vi "File Viewer v4.vi"() -> ()   [LabVIEW 2019]
uses:
  <vilib>/Utility/file.llb/Read Delimited Spreadsheet (I64).vi
  <vilib>/Utility/file.llb/Write Delimited Spreadsheet (DBL).vi
panel:
  in  "Stop":bool
  in  "Tab Control":T1(tab)
  in  "update":bool
  out "Raw Image From Camera":i32[][](graph)
  in  "File Path for Image:":path
  out "Expected position on spectrometer (pixels):":dbl
  in  "Grating:":u16(ring) items=["Shimadzu 30-006  "]
  in  "Laser:":u16(ring) items=["800nm  "]
  in  "Harmonic":dbl min=10.0 max=40.0
  out "l (nm)":dbl
  out "E (J)":dbl
  out "E (eV)":dbl
  out "Nearest Harmonic of 800nm":dbl
  out "Vertical Binned Waveform Graph":i64[](graph)
  out "Cursor Position (pixels)":dbl
  out "Distance to nearest harmonic of 800nm (pixels)":dbl
  in  "Caibration Date":u16(ring) items=["first calibration - 7/31", "7/31-current"]
  in  "Correct for QE?":bool
  in  "Save text file":bool
  in  "Graph to export:":u16(ring) items=["Wavelength Graph", "Energy Graph", "Harmonics Graph"]
  out "Wavelength Graph":T2(graph)
  out "Energy Graph (eV)":cluster{"eV":dbl, "QE scaled count":dbl}[](graph)
  out "Harmonics Graph":cluster{dbl, "QE scaled count":dbl}[](graph)
  in  "Pump/Probe Run Folder:":path
  out "Distance to nearest harmonic of 800nm (pixels)":dbl
  out "Cursor Position on CCD  (pixels)":dbl
  out "Nearest Harmonic of 800nm":dbl
  out "E (eV) 2":dbl
  out "E (J)":dbl
  out "l (nm)":dbl
  in  "Pump/Probe Harmonic:":dbl min=10.0 max=40.0
  out "Expected position on spectrometer (pixels):":dbl
  out "Time delay":dbl
  out "XUV":dbl[][](graph)
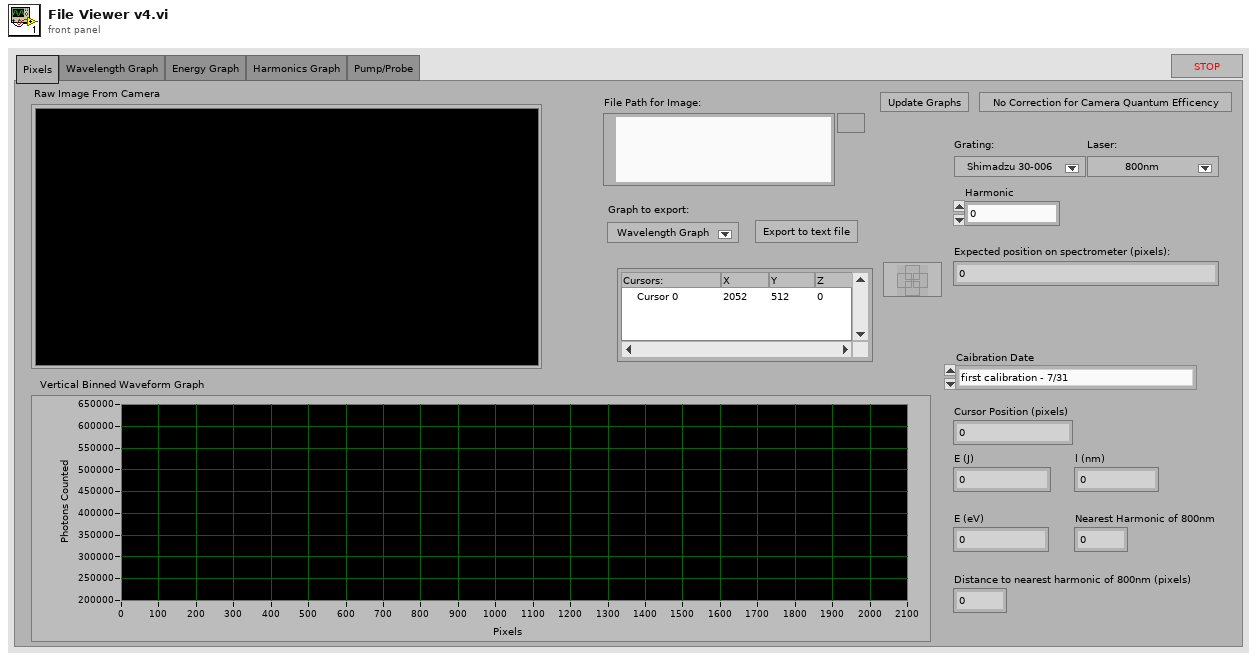
[diagram p1: front panel]
types:
  T1 = enum32{"Pixels", "Wavelength Graph", "Energy Graph", "Harmonics Graph", "Pump/Probe"}
  T2 = cluster{"No prefix":dbl, "QE scaled count":dbl}[]
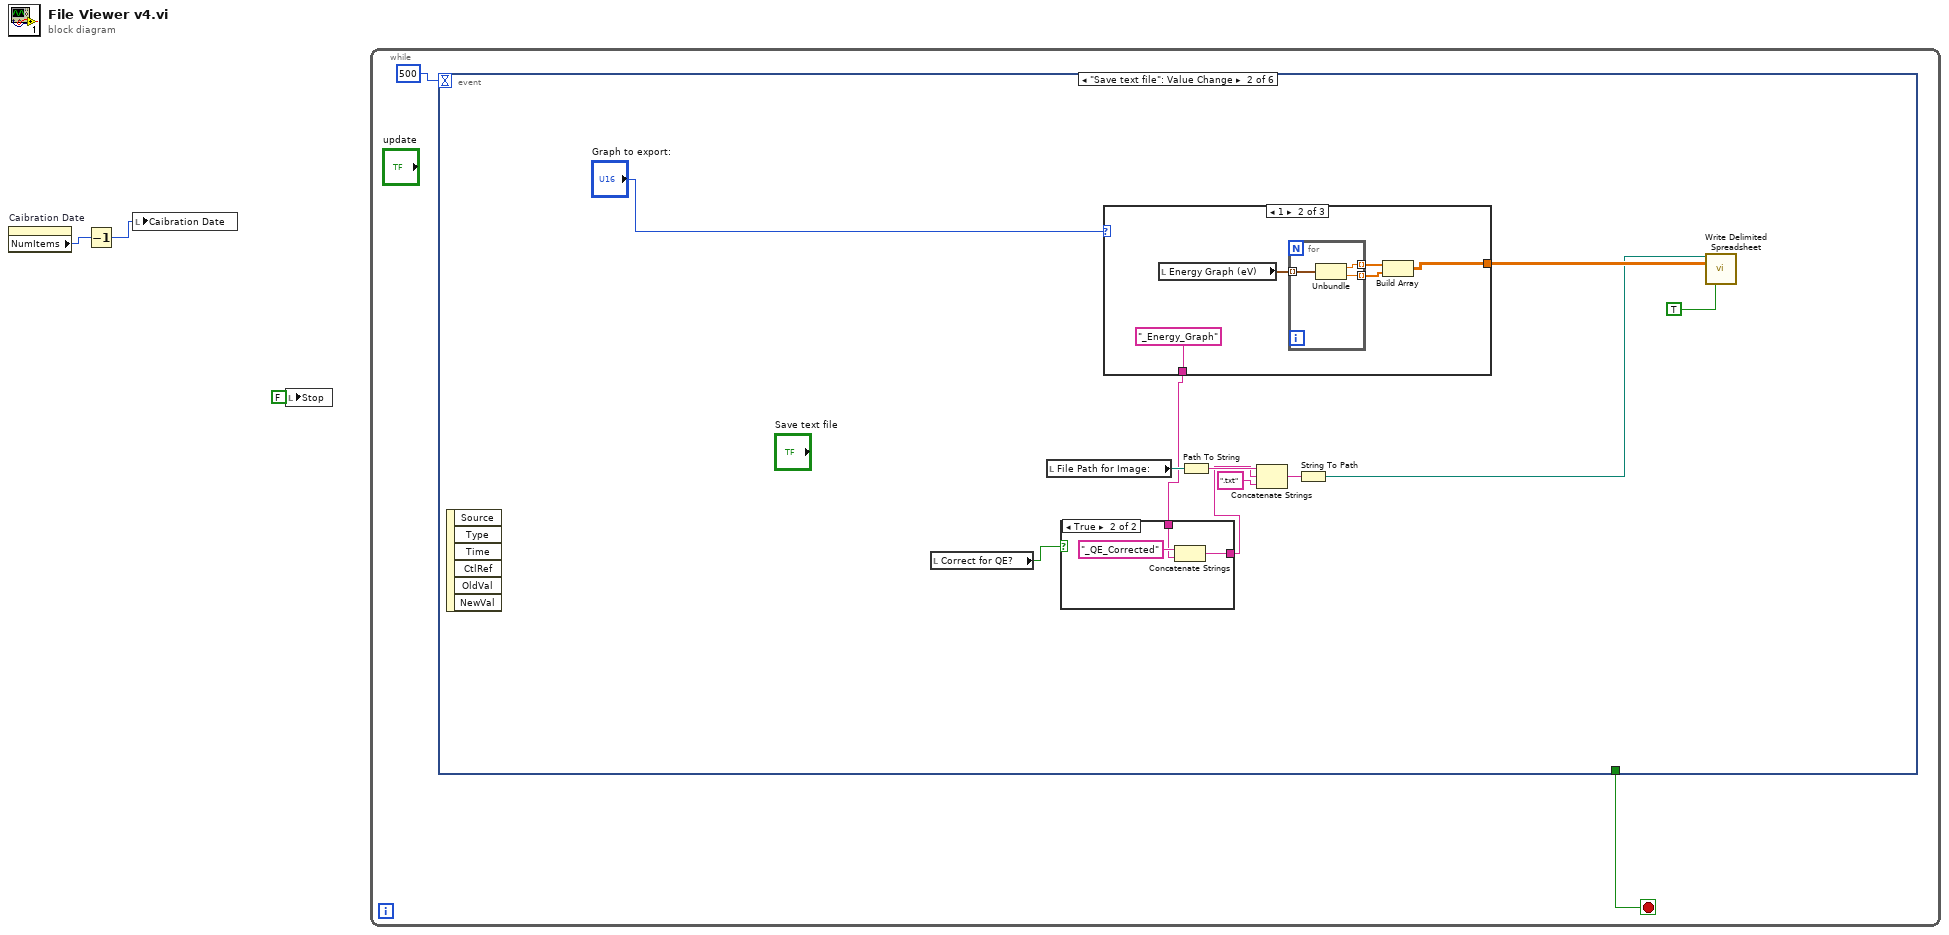
[diagram p0: block diagram]
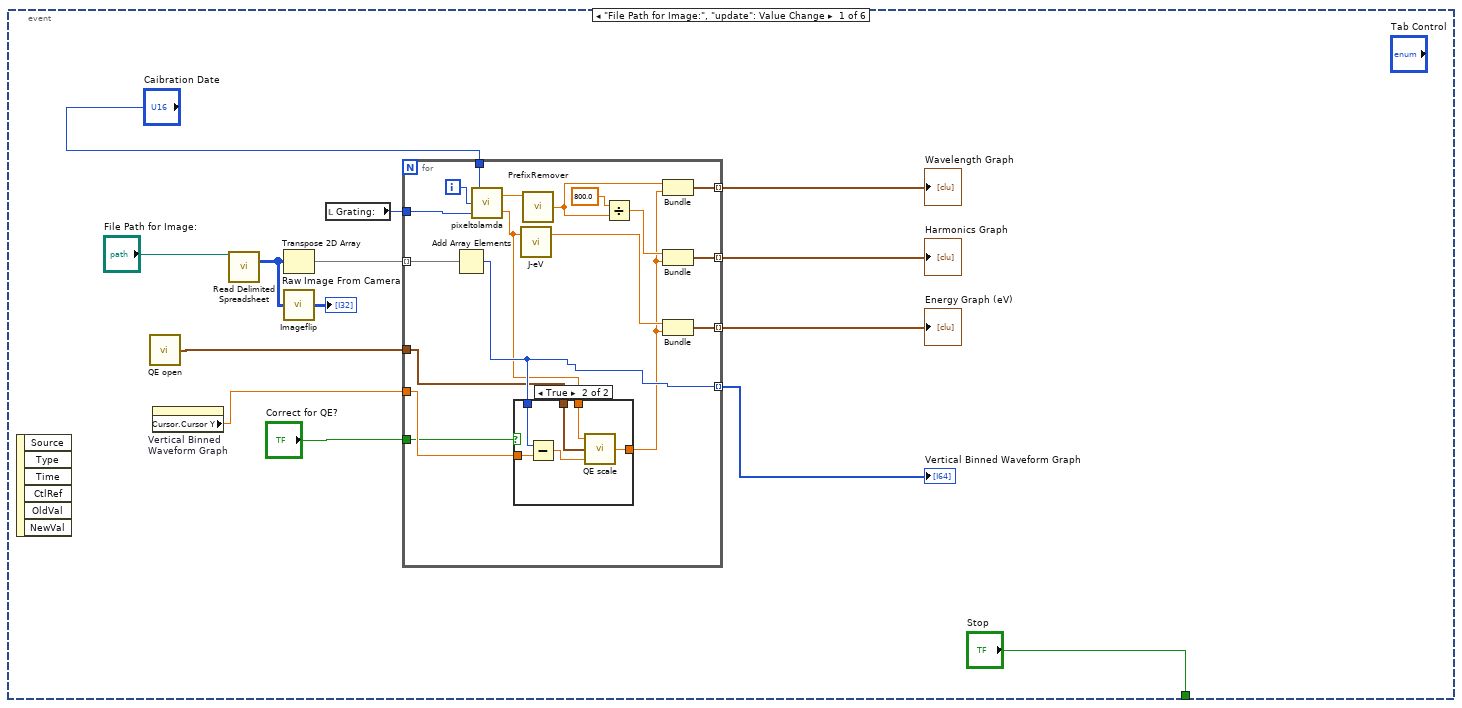
[diagram p2: hidden frame]
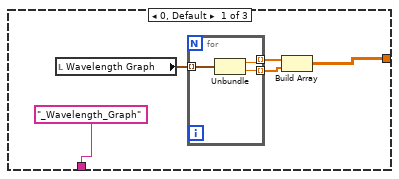
[diagram p5: hidden frame]
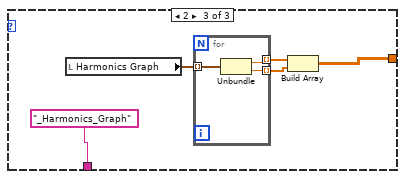
[diagram p6: hidden frame]
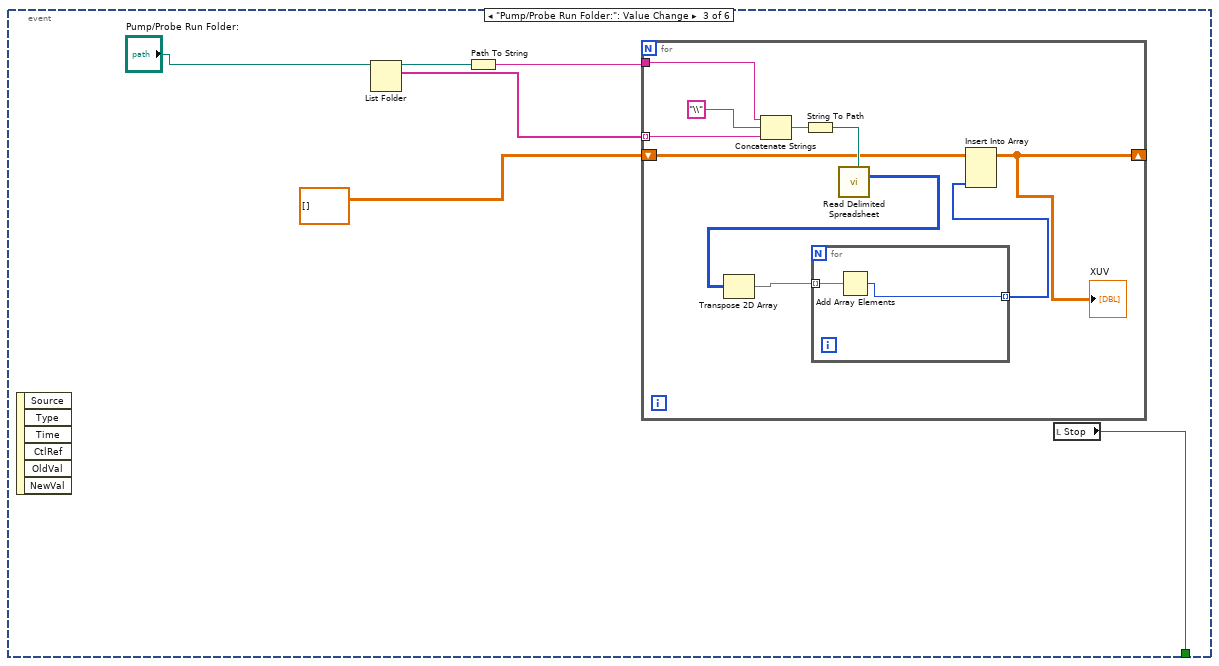
[diagram p7: hidden frame]
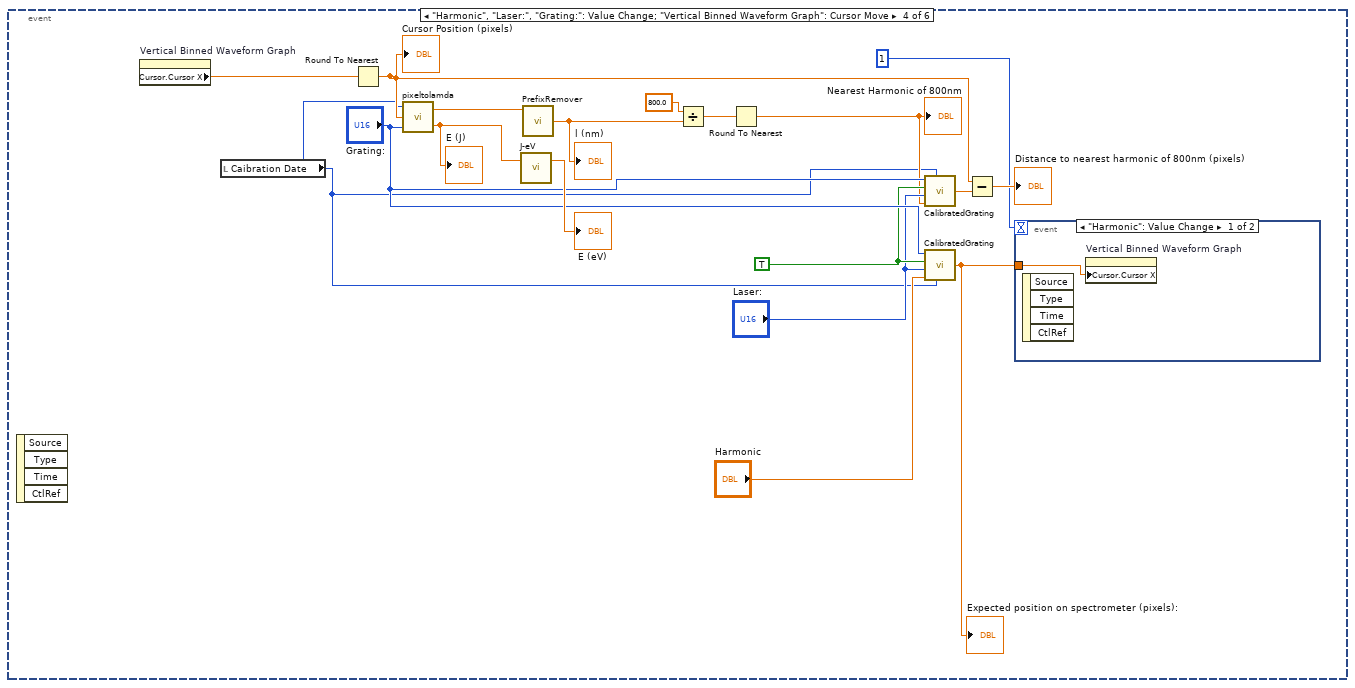
[diagram p8: hidden frame]
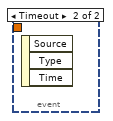
[diagram p9: hidden frame]
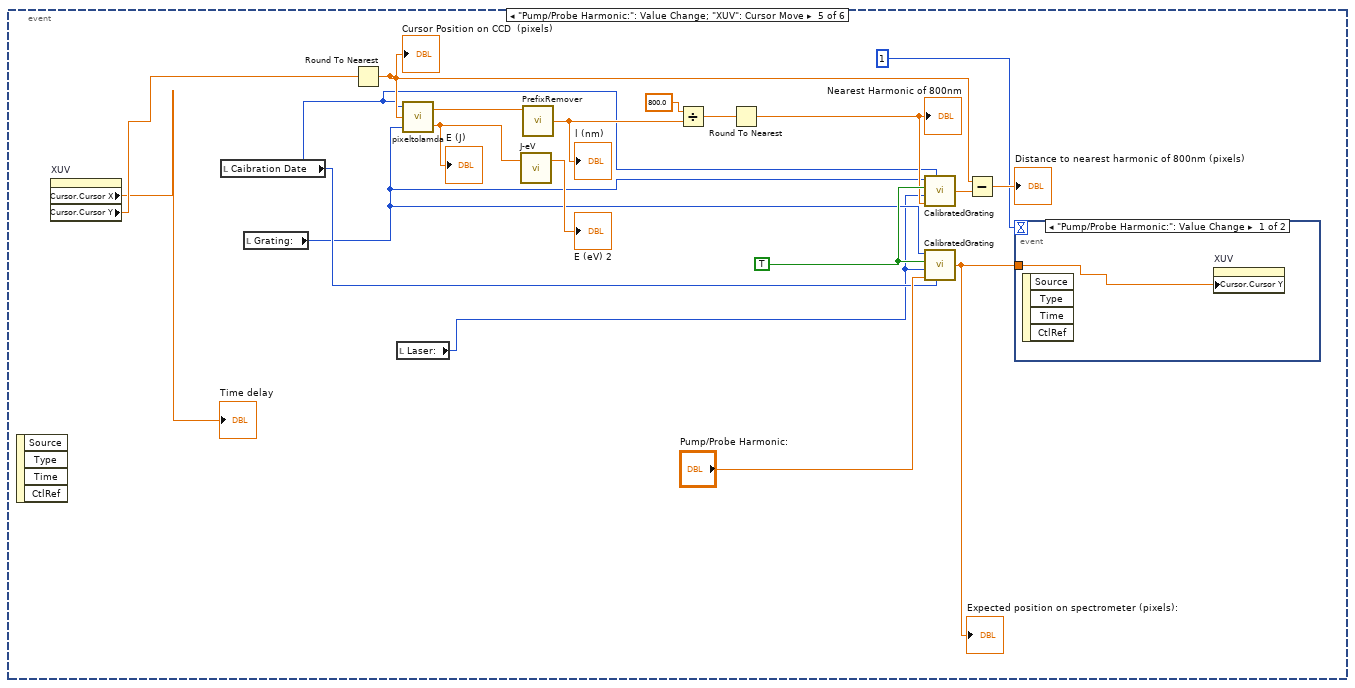
[diagram p10: hidden frame]
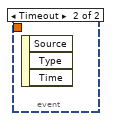
[diagram p11: hidden frame]
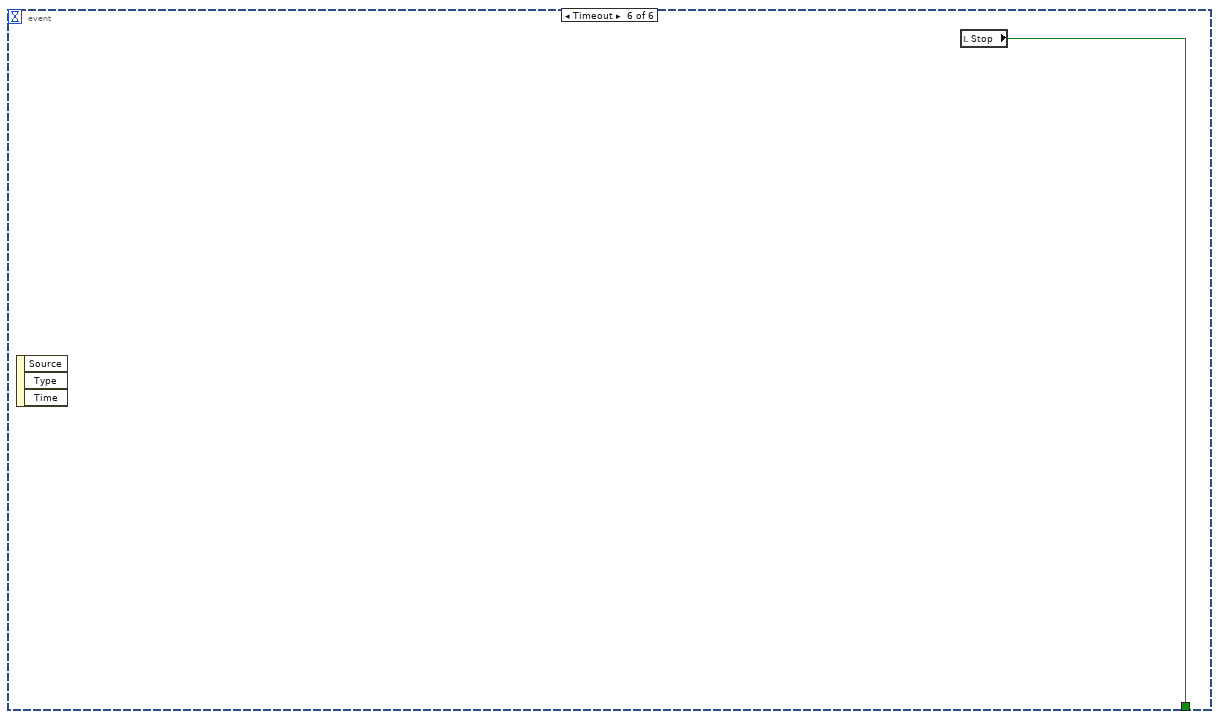
[diagram p12: hidden frame]
diagram:
  n1 = property on="Caibration Date" class="Ring (strict)"() -> ("NumItems"=w1:u32)  [unwired: 2 in, 2 out]
  n2 = Decrement(x=w1) -> (x-1=w2:u32)
  n3 = local write "Caibration Date"(w2) -> ()
  n4 = local write "Stop"(FALSE) -> ()
  n5 = while {
    stop <- w5 stop-if-true
    n6 = event shown="[1] \"Save text file\": Value Change" {
      selector: _ -> [_ _ _ _ _ _]
      dyn-events: _ -> [_ _ _ _ _ _]
      timeout: 500 -> [_ _ _ _ _ _]
      tunnel: ["Stop" _ w85 _ _ w141] -> w5
      event "File Path for Image:", "update": Value Change {
        n7 = event-data() -> ()  [unwired: 1 in, 6 out]
        n8 = call "QE open.vi"() -> ("QE data"=w8:cluster{"Numeric":dbl, dbl}[])
        n9 = property on="Vertical Binned Waveform Graph" class="WFGraph (strict)"() -> ("Cursor.Cursor Y"=w7:dbl)  [unwired: 2 in, 2 out]
        n10 = call-poly <vilib>:"Read Delimited Spreadsheet.vi"("file path (dialog if empty)"="File Path for Image:") -> ("all rows"=w16:i64[][])  [unwired: 9 in, 5 out]
        n11 = Transpose 2D Array(2D array=w16) -> (transposed array=w15:i64[][])
        n12 = call "Imageflip.vi"("2D array"=w16) -> ("transposed array"=→"Raw Image From Camera":i32[][])
        n13 = local read "Grating:"() -> (w13:u16)
        n14 = for {
          tunnel: w15 -> [w37] mode=indexing
          tunnel: [w25] -> w14 mode=indexing
          tunnel: w13 -> [w35]
          tunnel: [w34] -> w12 mode=indexing
          tunnel: [w33] -> w11 mode=indexing
          tunnel: [w28] -> w10 mode=indexing
          tunnel: "Caibration Date" -> [w27]
          tunnel: w8 -> [w24]
          tunnel: w7 -> [w26]
          tunnel: "Correct for QE?" -> [w21]
          i -> [w36]
          n15 = Add Array Elements(numeric array=w37) -> (sum=w25:i64)
          n16 = call "pixeltolamda.vi"("Grating:"=w35, "Pixel Postion"=w36, "Caibration Date"=w27) -> ("E (J)"=w20:dbl, "lamda (m)"=w31:dbl)
          n17 = case shown="True" w21 {
            tunnel: w26 -> [_ w44]
            tunnel: w25 -> [w38 w43]
            tunnel: w24 -> [_ w41]
            tunnel: w20 -> [_ w40]
            tunnel: [w38 w39] -> w22
            frame False {
            }
            frame True {
              n18 = Subtract(x=w43, y=w44) -> (x-y=w42:dbl)
              n19 = call "QE scale.vi"("Raw Photon Count"=w42, "QE data"=w41, "Energy (J)"=w40) -> ("QE scaled count"=w39:dbl)
            }
          }
          n20 = call "J-eV.vi"("J"=w20) -> ("eV"=w23:dbl)  [unwired: 1 in, 1 out]
          n21 = call "PrefixRemover.vi"("Nano"=w31) -> ("No prefix"=w30:dbl)  [unwired: 3 in]
          n22 = Divide(x=800.0, y=w30) -> (x/y=w29:dbl)
          n23 = Bundle("No prefix"=w30, "QE scaled count"=w22) -> (w34:cluster{"No prefix":dbl, "QE scaled count":dbl})  [unwired: 1 in]
          n24 = Bundle(w29, "QE scaled count"=w22) -> (w28:cluster{dbl, "QE scaled count":dbl})  [unwired: 1 in]
          n25 = Bundle("eV"=w23, "QE scaled count"=w22) -> (w33:cluster{"eV":dbl, "QE scaled count":dbl})  [unwired: 1 in]
        }
        "Vertical Binned Waveform Graph" <- w14
        "Wavelength Graph" <- w12
        "Energy Graph (eV)" <- w11
        "Harmonics Graph" <- w10
      }
      event "Save text file": Value Change {
        n26 = event-data() -> ()  [unwired: 1 in, 6 out]
        n27 = local read "Correct for QE?"() -> (w49:bool)
        n28 = local read "File Path for Image:"() -> (w52:path)
        n29 = case shown="1" "Graph to export:" {
          tunnel: [w61 w69 w77] -> w54
          tunnel: ["_Wavelength_Graph" ("pattern (all files)") "_Energy_Graph" ("pattern (all files)") "_Harmonics_Graph" ("pattern (all files)")] -> w47
          frame 0, Default {
            n30 = local read "Wavelength Graph"() -> (w64:T2)
            n31 = for {
              tunnel: w64 -> [w67] mode=indexing
              tunnel: [w66] -> w63 mode=indexing
              tunnel: [w65] -> w62 mode=indexing
              n32 = Unbundle(w67) -> ("No prefix"=w66:dbl, "QE scaled count"=w65:dbl)
            }
            n33 = Build Array(w63, w62) -> (w61:dbl[][])
          }
          frame 1 {
            n34 = local read "Energy Graph (eV)"() -> (w70:cluster{"eV":dbl, "QE scaled count":dbl}[])
            n35 = for {
              tunnel: w70 -> [w75] mode=indexing
              tunnel: [w74] -> w72 mode=indexing
              tunnel: [w73] -> w71 mode=indexing
              n36 = Unbundle(w75) -> ("eV"=w74:dbl, "QE scaled count"=w73:dbl)
            }
            n37 = Build Array(w72, w71) -> (w69:dbl[][])
          }
          frame 2 {
            n38 = local read "Harmonics Graph"() -> (w78:cluster{dbl, "QE scaled count":dbl}[])
            n39 = for {
              tunnel: w78 -> [w83] mode=indexing
              tunnel: [w82] -> w80 mode=indexing
              tunnel: [w81] -> w79 mode=indexing
              n40 = Unbundle(w83) -> (w82:dbl, "QE scaled count"=w81:dbl)
            }
            n41 = Build Array(w80, w79) -> (w77:dbl[][])
          }
        }
        n42 = case shown="True" w49 {
          tunnel: [w56 w58] -> w48
          tunnel: w47 -> [w56 w57]
          frame False {
          }
          frame True {
            n43 = Concatenate Strings("_QE_Corrected" ("pattern (all files)"), w57) -> (w58:string)
          }
        }
        n44 = Path To String(path=w52) -> (string=w51:string)
        n45 = Concatenate Strings(w51, w48, ".txt" ("pattern (all files)")) -> (w46:string)
        n46 = String To Path(string=w46) -> (path=w45:path)
        n47 = call-poly <vilib>:"Write Delimited Spreadsheet.vi"("file path (dialog if empty)"=w45, "2D data"=w54, "transpose? (no:F)"=TRUE) -> ()  [unwired: 11 in, 2 out]
      }
      event "Pump/Probe Run Folder:": Value Change {
        n48 = event-data() -> ()  [unwired: 1 in, 6 out]
        n49 = List Folder(path="Pump/Probe Run Folder:") -> (path out=w87:path, filenames=w88:string[])  [unwired: 3 in, 2 out]
        n50 = Path To String(path=w87) -> (string=w86:string)
        n51 = for {
          tunnel: w88 -> [w97] mode=indexing
          tunnel: w86 -> [w95]
          shift-right: [w90] -> _
          shift-left: dbl[][] [] -> [w94]
          n52 = Concatenate Strings(w95, "\\" ("string"), w97) -> (w99:string)
          n53 = String To Path(string=w99) -> (path=w98:path)
          n54 = call-poly <vilib>:"Read Delimited Spreadsheet.vi"("file path (dialog if empty)"=w98) -> ("all rows"=w92:i64[][])  [unwired: 9 in, 5 out]
          n55 = Transpose 2D Array(2D array=w92) -> (transposed array=w91:i64[][])
          n56 = for {
            tunnel: w91 -> [w101] mode=indexing
            tunnel: [w100] -> w93 mode=indexing
            n57 = Add Array Elements(numeric array=w101) -> (sum=w100:i64)
          }
          n58 = Insert Into Array(array=w94, new element=w93) -> (w90:dbl[][])  [unwired: 2 in]
          "XUV" <- w90
        }
        n59 = local read "Stop"() -> (w85:bool)
      }
      event "Harmonic", "Laser:", "Grating:": Value Change; "Vertical Binned Waveform Graph": Cursor Move {
        w111 = TRUE ("Subvi?")
        n60 = event-data() -> ()  [unwired: 1 in, 4 out]
        n61 = property on="Vertical Binned Waveform Graph" class="WFGraph (strict)"() -> ("Cursor.Cursor X"=w113:dbl)  [unwired: 2 in, 2 out]
        n62 = local read "Caibration Date"() -> (w102:u16)
        n63 = Round To Nearest(number=w113) -> (nearest integer value=w105:dbl)
        "Cursor Position (pixels)" <- w105
        n64 = call "pixeltolamda.vi"("Grating:"="Grating:", "Pixel Postion"=w105, "Caibration Date"=w102) -> ("E (J)"=w117:dbl, "lamda (m)"=w118:dbl)
        "E (J)" <- w117
        n65 = call "J-eV.vi"("J"=w117) -> ("eV"=→"E (eV)":dbl)  [unwired: 1 in, 1 out]
        n66 = call "PrefixRemover.vi"("Nano"=w118) -> ("No prefix"=w108:dbl)  [unwired: 3 in]
        "l (nm)" <- w108
        n67 = Divide(x=800.0, y=w108) -> (x/y=w115:dbl)
        n68 = Round To Nearest(number=w115) -> (nearest integer value=w109:dbl)
        "Nearest Harmonic of 800nm" <- w109
        n69 = call "CalibratedGrating.vi"("Grating:"="Grating:", "Subvi?"=w111, "Laser:"="Laser:", "Harmonic"=w109, "Caibration Date"=w102) -> ("Position on spectrometer (pixels):"=w107:dbl)
        n70 = call "CalibratedGrating.vi"("Grating:"="Grating:", "Subvi?"=w111, "Laser:"="Laser:", "Harmonic"="Harmonic", "Caibration Date"=w102) -> ("Position on spectrometer (pixels):"=w104:dbl)
        "Expected position on spectrometer (pixels):" <- w104
        n71 = Subtract(x=w105, y=w107) -> (x-y=→"Distance to nearest harmonic of 800nm (pixels)":dbl)
        n72 = event shown="[0] \"Harmonic\": Value Change" {
          selector: _ -> [_ _]
          dyn-events: _ -> [_ _]
          timeout: 1 -> [_ _]
          tunnel: w104 -> [w120 _]
          event "Harmonic": Value Change {
            n73 = event-data() -> ()  [unwired: 1 in, 4 out]
            n74 = property on="Vertical Binned Waveform Graph" class="WFGraph (strict)"("Cursor.Cursor X"=w120) -> ()  [unwired: 2 in, 2 out]
          }
          event Timeout {
            n75 = event-data() -> ()  [unwired: 1 in, 3 out]
          }
        }
      }
      event "Pump/Probe Harmonic:": Value Change; "XUV": Cursor Move {
        w133 = TRUE ("Subvi?")
        n76 = event-data() -> ()  [unwired: 1 in, 4 out]
        n77 = property on="XUV" class="IntGraph (strict)"() -> ("Cursor.Cursor X"=→"Time delay":dbl, "Cursor.Cursor Y"=w122:dbl)  [unwired: 2 in, 2 out]
        n78 = local read "Caibration Date"() -> (w125:u16)
        n79 = local read "Grating:"() -> (w124:u16)
        n80 = Round To Nearest(number=w122) -> (nearest integer value=w128:dbl)
        "Cursor Position on CCD  (pixels)" <- w128
        n81 = local read "Laser:"() -> (w123:u16)
        n82 = call "pixeltolamda.vi"("Grating:"=w124, "Pixel Postion"=w128, "Caibration Date"=w125) -> ("E (J)"=w137:dbl, "lamda (m)"=w138:dbl)
        "E (J)" <- w137
        n83 = call "J-eV.vi"("J"=w137) -> ("eV"=→"E (eV) 2":dbl)  [unwired: 1 in, 1 out]
        n84 = call "PrefixRemover.vi"("Nano"=w138) -> ("No prefix"=w131:dbl)  [unwired: 3 in]
        "l (nm)" <- w131
        n85 = Divide(x=800.0, y=w131) -> (x/y=w135:dbl)
        n86 = Round To Nearest(number=w135) -> (nearest integer value=w132:dbl)
        "Nearest Harmonic of 800nm" <- w132
        n87 = call "CalibratedGrating.vi"("Grating:"=w124, "Subvi?"=w133, "Laser:"=w123, "Harmonic"=w132, "Caibration Date"=w125) -> ("Position on spectrometer (pixels):"=w130:dbl)
        n88 = call "CalibratedGrating.vi"("Grating:"=w124, "Subvi?"=w133, "Laser:"=w123, "Harmonic"="Pump/Probe Harmonic:", "Caibration Date"=w125) -> ("Position on spectrometer (pixels):"=w127:dbl)
        "Expected position on spectrometer (pixels):" <- w127
        n89 = Subtract(x=w128, y=w130) -> (x-y=→"Distance to nearest harmonic of 800nm (pixels)":dbl)
        n90 = event shown="[0] \"Pump/Probe Harmonic:\": Value Change" {
          selector: _ -> [_ _]
          dyn-events: _ -> [_ _]
          timeout: 1 -> [_ _]
          tunnel: w127 -> [w140 _]
          event "Pump/Probe Harmonic:": Value Change {
            n91 = event-data() -> ()  [unwired: 1 in, 4 out]
            n92 = property on="XUV" class="IntGraph (strict)"("Cursor.Cursor Y"=w140) -> ()  [unwired: 2 in, 2 out]
          }
          event Timeout {
            n93 = event-data() -> ()  [unwired: 1 in, 3 out]
          }
        }
      }
      event Timeout {
        n94 = event-data() -> ()  [unwired: 1 in, 3 out]
        n95 = local read "Stop"() -> (w141:bool)
      }
    }
  }
